vi "Create Channels.vi"(8 "error in (no error)":errorcluster, 10 "9224 in":refnum<class "9224.lvclass">, 11 "Parent Ref in":T1 format="%.0x") -> (0 "error out":errorcluster, 2 "9224 out":refnum<class "9224.lvclass">, 3 "Parent Ref out":T1 format="%.0x")   [LabVIEW 2017, in "Modules.lvlib" / "9224.lvclass"]
uses:
  9224.lvclass
  <vilib>/NI Veristand/Custom Device API/Custom Device Item Ref.ctl
  RSI Module/RSI Module.lvclass
  <vilib>/NI Veristand/Custom Device API/Custom Device API.lvlib
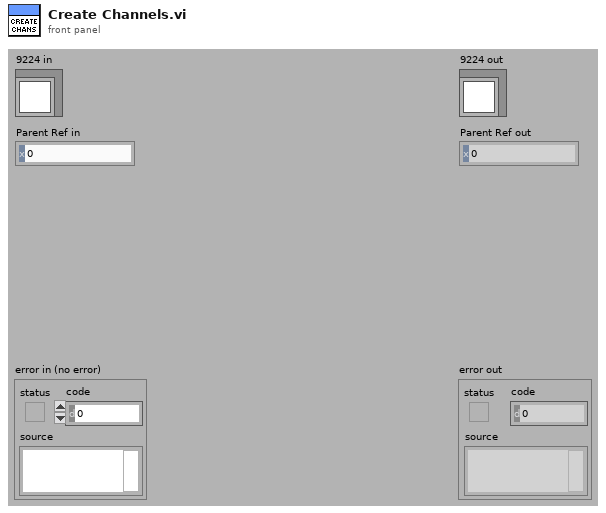
[diagram p1: front panel]
types:
  T1 = typedef "Custom Device API.lvlib/Custom Device Item Ref.ctl" = u64
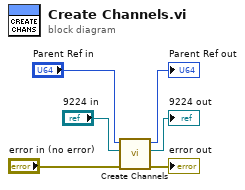
[diagram p0: block diagram]
diagram:
  n1 = call-parent "Create Channels.vi"("error in (no error)"="error in (no error)", "RSI Module in"="9224 in", "Parent Ref in"="Parent Ref in") -> ("error out"=→"error out":errorcluster, "RSI Module out"=→"9224 out":refnum<class "9224.lvclass">, "Parent Ref out"=→"Parent Ref out":T1)  [unwired: 6 in]
